vi "Analog Input - 1 Channel - 1 Sample.vi"() -> ()   [LabVIEW 2019]
uses:
  <vilib>/myRIO/Instrument Drivers/Onboard IO/AI/typedefs/AI Reference.ctl
  <vilib>/myRIO/Common/Instrument Driver Framework/Utilities/typedefs/myRIO Generic Hardware Reference.ctl
  <vilib>/myRIO/Common/Instrument Driver Framework/Utilities/typedefs/Hardware Version Enum.ctl
  <vilib>/myRIO/Common/Instrument Driver Framework/Utilities/typedefs/myRIO v1.0 Reference.ctl
  <vilib>/myRIO/Common/Instrument Driver Framework/Utilities/typedefs/Generic FPGA Reference.ctl
  <vilib>/myRIO/Common/Instrument Driver Framework/myRIO v1.0/AI/typedefs/AI Channels List.ctl
  <vilib>/myRIO/Common/Instrument Driver Framework/myRIO v1.0/AI/typedefs/AI Channels Enum.ctl
  <vilib>/myRIO/Common/Instrument Driver Framework/Utilities/typedefs/Analog Scaling Constants List.ctl
  <vilib>/myRIO/Common/Instrument Driver Framework/Utilities/typedefs/Analog Scaling Constants.ctl
  <vilib>/userdefined/High Color/nirio_resource_hc.ctl
  <vilib>/myRIO/Common/Instrument Driver Framework/Utilities/vis/Is FPGA Ref Available.vi
  <vilib>/myRIO/Common/Instrument Driver Framework/ELVIS III v1.0/AI/vis/ELVIS III v1.1 Open AI.vi
  <vilib>/myRIO/Instrument Drivers/Onboard IO/AI/vis/Read.vi
  <vilib>/myRIO/Common/Instrument Driver Framework/Utilities/vis/Validate Channels.vi
  <vilib>/myRIO/Common/Instrument Driver Framework/ELVIS III v1.0/AI/vis/ELVIS III v1.0 Reserve AI.vi
  <vilib>/myRIO/Common/Instrument Driver Framework/myRIO v1.0/UART/vis/myRIO v1.0 Close UART.vi
  <vilib>/myRIO/Common/Instrument Driver Framework/ELVIS III v1.0/AI/vis/ELVIS III v1.0 Build MUX Configuration AI.vi
  <vilib>/Utility/VariantDataType/GetNumericInfo.vi
  <vilib>/Utility/error.llb/Error Cluster From Error Code.vi
  <vilib>/myRIO/Common/Instrument Driver Framework/ELVIS III v1.0/ELVIS III v1.1 Open.vi
  <vilib>/myRIO/Common/Instrument Driver Framework/ELVIS III v1.0/Resource Manager/vis/ELVIS III v1.0 Coerce AI Scaling.vi
  <vilib>/myRIO/Common/Instrument Driver Framework/ELVIS III v1.0/Resource Manager/vis/ELVIS III v1.0 Reserve Channel List.vi
  <vilib>/myRIO/Common/Instrument Driver Framework/ELVIS III v1.0/Resource Manager/vis/ELVIS III v1.0 Configure AI Mode.vi
  <vilib>/myRIO/Common/Instrument Driver Framework/myRIO v1.0/myRIO v1.0 Close.vi
  <vilib>/myRIO/Common/Instrument Driver Framework/ELVIS III v1.0/AI/vis/ELVIS III v1.0 Read AI.vi
  <vilib>/myRIO/Common/Instrument Driver Framework/Utilities/vis/FPGA Ref Manager.vi
  <vilib>/myRIO/Common/Instrument Driver Framework/ELVIS III v1.0/ELVIS III v1.0 Reset FPGA.vi
  <vilib>/myRIO/Common/Instrument Driver Framework/myRIO v1.0/IRQ/vis/myRIO v1.0 IRQ Info FGV.vi
  <vilib>/myRIO/Common/Instrument Driver Framework/myRIO v1.0/IRQ/vis/myRIO v1.0 Timer IRQ Info FGV.vi
  <vilib>/myRIO/Common/Instrument Driver Framework/myRIO v1.0/IRQ/vis/myRIO v1.0 ISR Agent.vi
  <vilib>/myRIO/Instrument Drivers/Utilities/vis/Reset Index.vi
  <vilib>/myRIO/Common/Instrument Driver Framework/myRIO v1.0/Resource Manager/vis/myRIO v1.0 Block Write Resource Manager.vi
  <vilib>/myRIO/Express VI/Onboard IO/AI/AI Express VI.xnode
  <vilib>/myRIO/Instrument Drivers/Onboard IO/AI/vis/myRIO AI Open.xnode
  <vilib>/myRIO/Instrument Drivers/Onboard IO/AI/AI.lvlib
  <vilib>/myRIO/Instrument Drivers/Utilities/Utilities.lvlib
panel:
  out "Analog Data":dbl(graph)
  in  "Stop":bool
  # "ELVIS III Control IO"
  # "模拟输入单通道单采样"
  # "Overview: Acquires single point voltage values each loop iteration from Bank A, Channel 0 (A/AI0).\nInstructions:\n1. Connect A/AI0 to a valid signal.\n2. Run the VI."
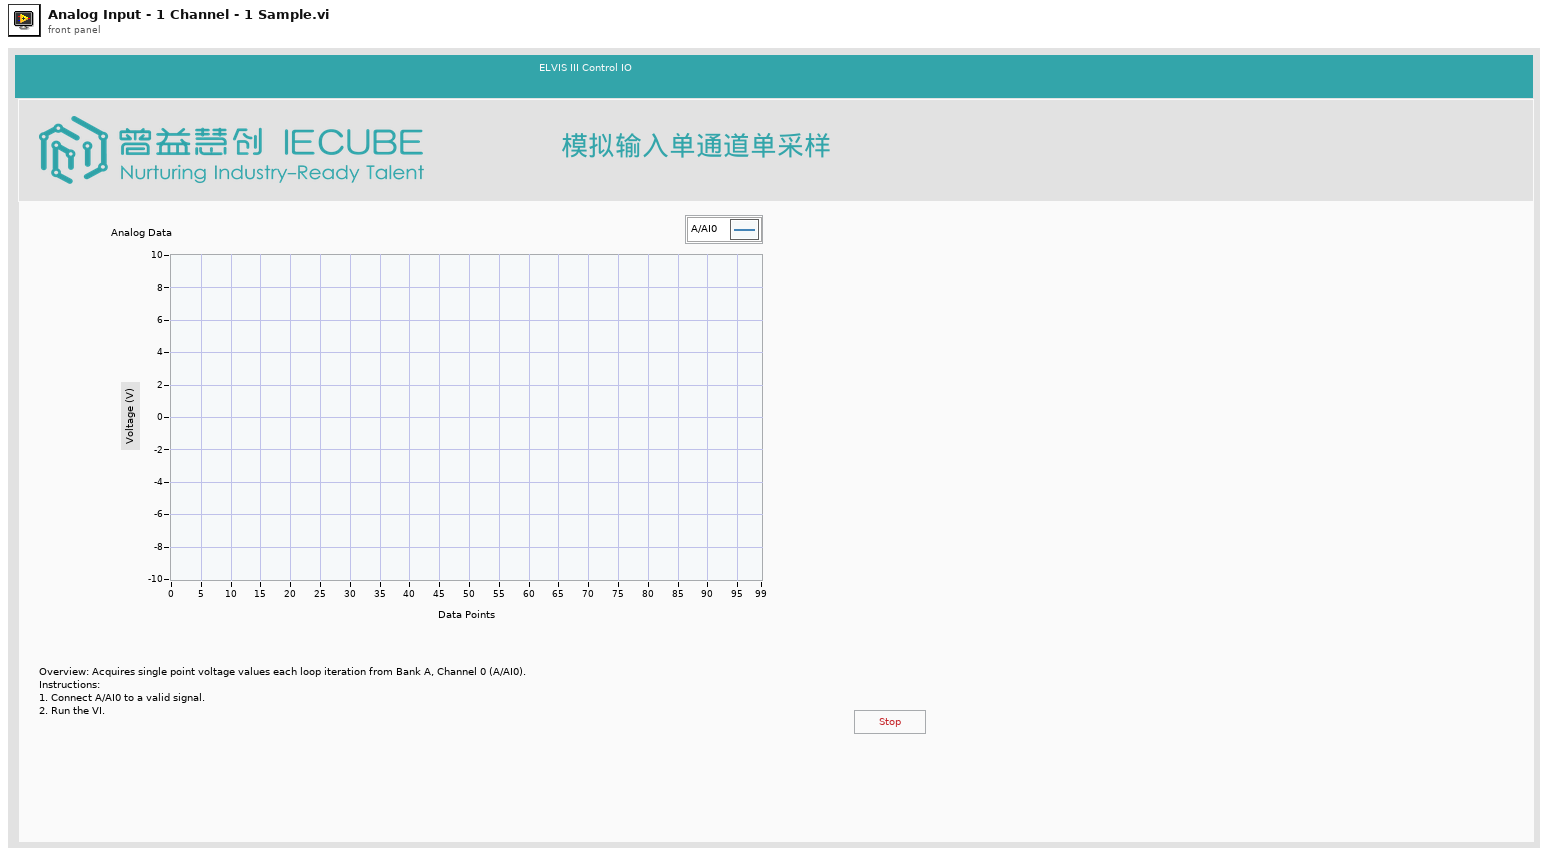
[diagram p1: front panel]
types:
  T1 = typedef "AI.lvlib/AI Reference.ctl" = cluster{"myRIO Reference":T2, "AI Channels List":T6, "AI Scaling Constants List":T8}
  T2 = typedef "myRIO Generic Hardware Reference.ctl" = cluster{"myRIO Model":T3, "myRIO Hardware Reference":T4}
  T3 = typedef "Hardware Version Enum.ctl" = enum16{"Unknown", "myRIO-1900", "myRIO-1950", "roboRIO", "NI ELVIS RIO CM", "ELVIS III"}
  T4 = typedef "myRIO v1.0 Reference.ctl" = cluster{"Generic FPGA Reference":T5, "Allow multiple opens":bool}
  T5 = typedef "Generic FPGA Reference.ctl" = refnum<k20>
  T6 = typedef "AI Channels List.ctl" = T7[]
  T7 = typedef "AI Channels Enum.ctl" = enum16{"Not Connected", "AudioIn/Left", "AudioIn/Right", "C/AI0", "C/AI1", "A/AI0", "A/AI1", "A/AI2", "A/AI3", "A/AI4", "A/AI5", "A/AI6", "A/AI7", "B/AI0", "B/AI1", "B/AI2", "B/AI3", "B/AI4", "B/AI5", "B/AI6", "B/AI7", "AI/AI0", "AI/AI1", "AI/AI2", "AI/AI3", "A/AI0 (DIFF)", "A/AI1 (DIFF)", "A/AI2 (DIFF)", "A/AI3 (DIFF)", "B/AI0 (DIFF)", "B/AI1 (DIFF)", "B/AI2 (DIFF)", "B/AI3 (DIFF)"}
  T8 = typedef "Analog Scaling Constants List.ctl" = T9[]
  T9 = typedef "Analog Scaling Constants.ctl" = cluster{"LSB Weight (Volts)":dbl, "Offset (Volts)":dbl, "Signed?":bool}
  T10 = typedef "nirio_resource_hc.ctl" = tag
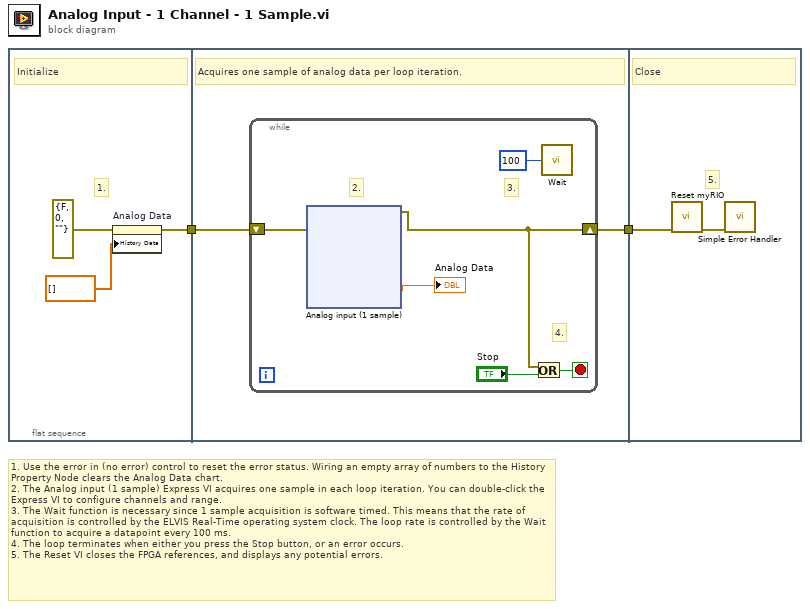
[diagram p0: block diagram]
diagram:
  # "1. Use the error in (no error) control to reset the error status. Wiring an empty array of numbers to the History Property Node clears the Analog Data chart.\n2. The Analog input (1 sample) Express VI acquires one sample in each loop iteration. You can double-click the Express VI to configure channels and range.\n3. The Wait function is necessary since 1 sample acquisition is software timed. This means that the rate of acquisition is controlled by the ELVIS Real-Time operating system clock. The loop rate is controlled by the Wait function to acquire a datapoint every 100 ms.\n4. The loop terminates when either you press the Stop button, or an error occurs.\n5. The Reset VI closes the FPGA references, and displays any potential errors."
  n1 = flat-sequence {
    tunnel: [w5] -> w2
    tunnel: w2 -> [w7]
    tunnel: [w6] -> w1
    tunnel: w1 -> [w58]
    frame #0 {
      # "1."
      # "Initialize"
      n2 = property on="Analog Data" class="WFChart (严格)"(error in=errorcluster {"status"=FALSE, "code"=0, "source"=""} ("error in (no error)"), "History Data"=dbl[] []) -> (error out=w5:errorcluster)  [unwired: 1 in, 1 out]
    }
    frame #1 {
      # "Acquires one sample of analog data per loop iteration."
      n3 = while {
        shift-right: [w11] -> w6
        shift-left: w7 -> [w13]
        stop <- w12 stop-if-true
        # "4."
        # "3."
        # "2."
        n4 = xnode "Analog input (1 sample)"("error in (no error)"=w13) -> ("A/AI0"=→"Analog Data":dbl, "error out"=w11:errorcluster)
        n5 = Or(x=w11, y="Stop") -> (x .or. y?=w12:bool)
        n6 = call "Wait"("Count(mSec)"=u32 100) -> ()  [unwired: 1 out]
      }
    }
    frame #2 {
      # "5."
      # "Close"
      n7 = call <vilib>:"Reset myRIO.vi"("error in (no error)"=w58) -> ("error out"=w57:errorcluster)  [unwired: 10 in]
      n8 = call <vilib>:"Simple Error Handler.vi"("error in (no error)"=w57) -> ()  [unwired: 4 in, 5 out]
    }
  }
